vi "Insert Element.vi"(0 "Session Handle in":T1, 5 "Value":dbl, 11 "error in (no error)":errorcluster) -> (4 "Session Handle out":T1, 15 "error out":errorcluster)   [LabVIEW 2015, in "Circular Buffer.lvclass"]
uses:
  Circular Buffer.lvclass
  Typedefs/Session Handle.ctl
  Circular Buffer.lvclass/Circular Buffer.ctl
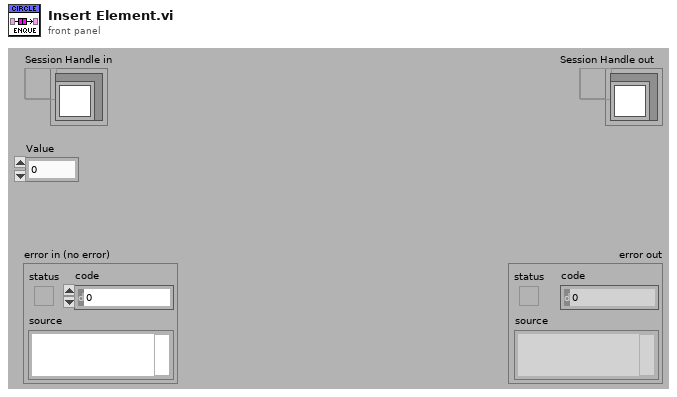
[diagram p1: front panel]
types:
  T1 = typedef "Circular Buffer.lvclass/Session Handle.ctl" = refnum<data-value>
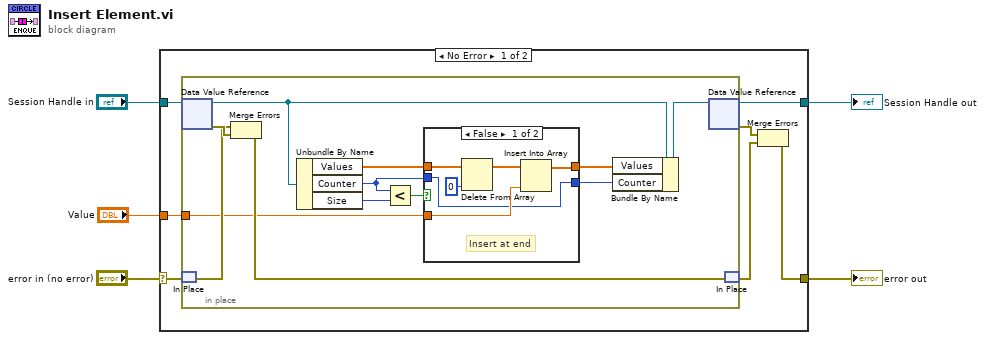
[diagram p0: block diagram]
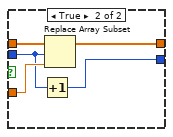
[diagram p2: hidden frame]
diagram:
  n1 = case shown="No Error" "error in (no error)" {
    selector: "error in (no error)" -> [w7 w36]
    tunnel: "Session Handle in" -> [w12 w37]
    tunnel: [w11 w37] -> w4
    tunnel: [w8 w36] -> w3
    tunnel: "Value" -> [w6 _]
    frame No Error {
      n2 = in-place {
        in-place-border: w6 -> [w15]
        n3 = in-place-dvr #1(w12) -> (w20:refnum<class "Circular Buffer.lvclass">, w23:errorcluster)
        n4 = in-place-match #2(w7) -> (w22:errorcluster)
        n5 = Merge Errors(w22, w23) -> (w24:errorcluster)
        n6 = Unbundle By Name(w20) -> ("Values"=w17:dbl[], "Counter"=w16:u16, "Size"=w19:u16)
        n7 = Less?(x=w16, y=w19) -> (x < y?=w18:bool)
        n8 = case shown="False" w18 {
          tunnel: w17 -> [w30 w35]
          tunnel: w16 -> [w26 w32]
          tunnel: w15 -> [w27 w34]
          tunnel: [w25 w33] -> w14
          tunnel: [w26 w31] -> w13
          frame False {
            # "Insert at end"
            n9 = Delete From Array(array=w30, index=0) -> (array with subset deleted=w28:dbl[])  [unwired: 1 in, 1 out]
            n10 = Insert Into Array(array=w28, new element=w27) -> (w25:dbl[])  [unwired: 1 in]
          }
          frame True {
            n11 = Increment(x=w32) -> (x+1=w31:u16)
            n12 = Replace Array Subset(array=w35, new element=w34, index=w32) -> (w33:dbl[])
          }
        }
        n13 = Bundle By Name(cluster=w20, "Values"=w14, "Counter"=w13) -> (w21:refnum<class "Circular Buffer.lvclass">)
        n14 = in-place-dvr #1(w21) -> (w11:T1, w9:errorcluster)
        n15 = in-place-match #2(w24) -> (w10:errorcluster)
      }
      n16 = Merge Errors(w9, w10) -> (w8:errorcluster)
    }
    frame Error {
    }
  }
  "Session Handle out" <- w4
  "error out" <- w3
